vi "while_v0_v12.vi"() -> ()   [LabVIEW 2009]
panel:
  in  "A_max":dbl(slide)=63.905325443786985 scale=0.0..100.0
  in  "Delay":dbl(slide)=21.714285714285715 scale=10.0..100.0
  out "Waveform Chart":i64(graph)=58
  out "Ampl":i64=58
  in  "Panta":i64(knob)=2 scale=0.0..10.0
  in  "stop":bool
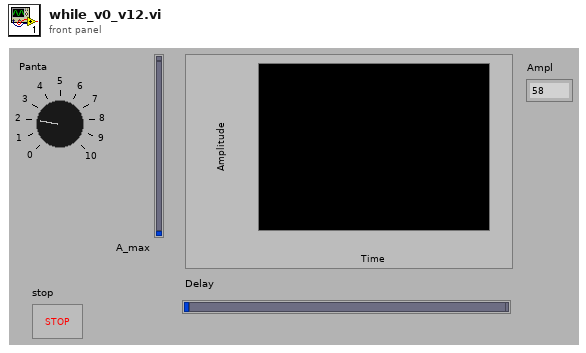
[diagram p1: front panel]
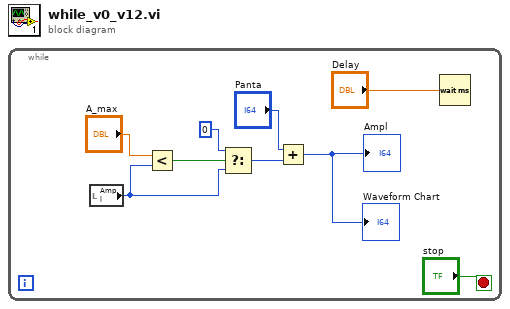
[diagram p0: block diagram]
diagram:
  n1 = while {
    stop <- "stop" stop-if-true
    n2 = local read "Ampl"() -> (w5:i64)
    n3 = Less?(x="A_max", y=w5) -> (x < y?=w7:bool)
    n4 = Select(t=i64 0, s=w7, f=w5) -> (s? t:f=w4:i64)
    n5 = Add(x="Panta", y=w4) -> (x+y=→"Ampl" →"Waveform Chart":i64)
    n6 = Wait (ms)(milliseconds to wait="Delay") -> ()  [unwired: 1 out]
  }
